vi "Set Control Parameters.vi"(8 "error in (no error)":errorcluster, 10 "Control Parameters":T1 {"Default Range" items=["Off", "Low (0.5W)", "Med (5W)", "High (50W)"]; "Heater Range" items=["Off", "Low (0.5W)", "Med (5W)", "High (50W)"]; "Manual Power (%)" format="%.3f"; "Mode" items=["Manual PID"=1, "Zone"=2, "Open Loop"=3, "AutoTune PID"=4, "AutoTune PI"=5, "AutoTune P"=6]}, 11 "Lakeshore 331 in":refnum<class "Lakeshore 331.lvclass">) -> (0 "error out":errorcluster, 3 "Lakeshore 331 out":refnum<class "Lakeshore 331.lvclass">)   [LabVIEW 2022 SP3, in "Lakeshore 331.lvclass"]
uses:
  Lakeshore 331.lvclass
  Temp Control Parameters.ctl
  Lakeshore 331.lvclass/Lakeshore 331.ctl
  Temp Control.lvclass
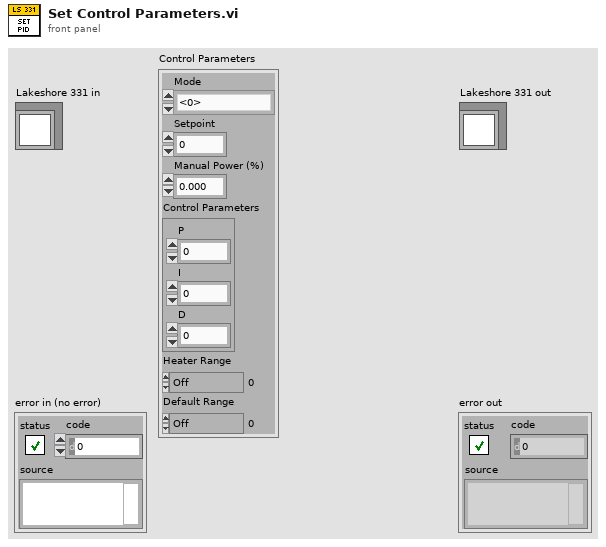
[diagram p1: front panel]
types:
  T1 = typedef "Temp Control.lvclass/Temp Control Parameters.ctl" = cluster{"Mode":u16, "Setpoint":dbl, "Manual Power (%)":dbl, "Control Parameters":cluster{"P":dbl, "I":dbl, "D":u16}, "Heater Range":u16, "Default Range":u16}
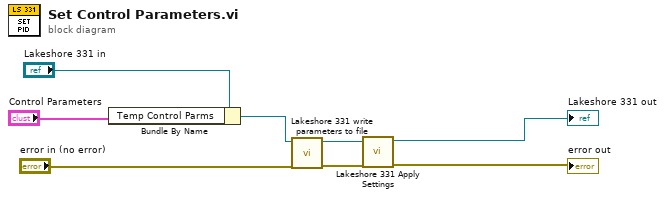
[diagram p0: block diagram]
diagram:
  n1 = Bundle By Name(cluster="Lakeshore 331 in", "Temp Control Parms"="Control Parameters") -> (w6:refnum<class "Lakeshore 331.lvclass">)
  n2 = call "Lakeshore 331 write parameters to file.vi"("error in (no error)"="error in (no error)", "Lakeshore 331 in"=w6) -> ("error out"=w2:errorcluster, "Lakeshore 331 out"=w5:refnum<class "Lakeshore 331.lvclass">)  [unwired: 8 in]
  n3 = call "Lakeshore 331 Apply Settings.vi"("error in (no error)"=w2, "Lakeshore 331 in"=w5) -> ("error out"=→"error out":errorcluster, "Lakeshore 331 out"=→"Lakeshore 331 out":refnum<class "Lakeshore 331.lvclass">)  [unwired: 8 in]
